vi "setState0ByFile.vi"(8 "error in (no error)":errorcluster, 10 "State 0 File Name":string="state0inDof.txt", 11 "OptCtrl in":refnum<class "OptCtrl.lvclass">) -> (0 "error out":errorcluster, 3 "OptCtrl out":refnum<class "OptCtrl.lvclass">)   [LabVIEW 2016, in "OptCtrl.lvclass"]
doc: "Set the state 0 (x0) in degree of freedom (DOF) based on the file."
uses:
  OptCtrl.lvclass
  OptCtrl.lvclass/OptCtrl.ctl
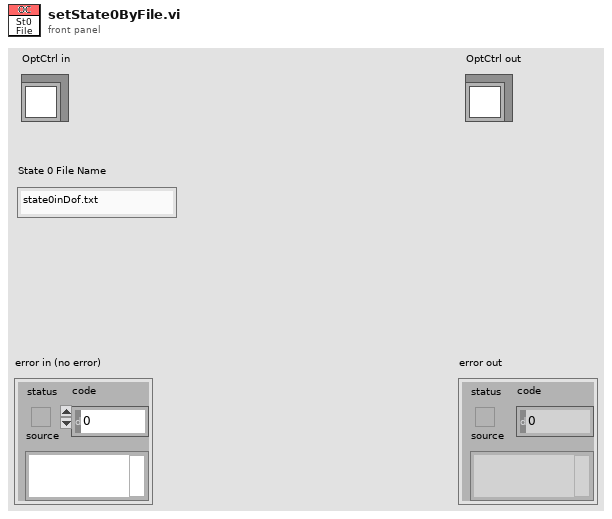
[diagram p1: front panel]
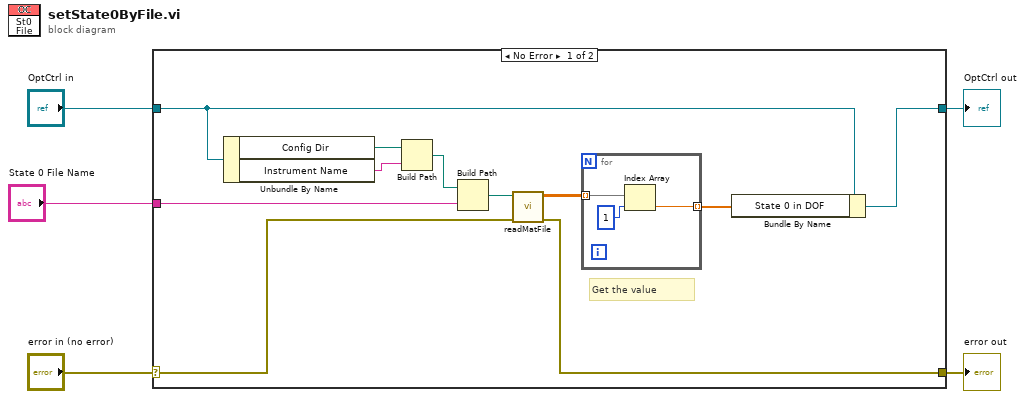
[diagram p0: block diagram]
diagram:
  n1 = case shown="No Error" "error in (no error)" {
    selector: "error in (no error)" -> [w12 w21]
    tunnel: [w11 w21] -> w4
    tunnel: [w6 w20] -> w2
    tunnel: "OptCtrl in" -> [w7 w20]
    tunnel: "State 0 File Name" -> [w13 _]
    frame No Error {
      # "Get the value"
      n2 = Unbundle By Name(w7) -> ("Config Dir"=w16:path, "Instrument Name"=w15:string)
      n3 = Build Path(base path=w16, name or relative path=w15) -> (appended path=w14:path)
      n4 = Build Path(base path=w14, name or relative path=w13) -> (appended path=w10:path)
      n5 = call "readMatFile.vi"("error in (no error)"=w12, "Path"=w10) -> ("error out"=w11:errorcluster, "Matrix"=w9:dbl[][])  [unwired: 8 in]
      n6 = for {
        tunnel: w9 -> [w19] mode=indexing
        tunnel: [w17] -> w8 mode=indexing
        n7 = Index Array(array=w19, index=1) -> (element=w17:dbl)
      }
      n8 = Bundle By Name(cluster=w7, "State 0 in DOF"=w8) -> (w6:refnum<class "OptCtrl.lvclass">)
    }
    frame Error {
    }
  }
  "error out" <- w4
  "OptCtrl out" <- w2
